vi "1.2.1-ParseYPR.vi"(9 "ASCII: VNYPR,":u8[](array[numeric])=[86, 78, 89, 80, 82, 44], 10 "Serial Byte":u8) -> (1 "Yaw":i16)   [LabVIEW 2010]
doc: "This VI parses Yaw, Pitch, and Roll (YPR) data from the VectorNav. In response to a YPR Read Request, the VectorNav will reply in the form \"$VNYPR,XX,-XXX.XX,-XXX.XX,+XXX.XX*XX\" (where X is a digit from 0-9). This string is in the form \"$<command type>,<access ID>, <yaw>,<pitch>,<roll>\".\n\nThe VI first waits for a $, then checks to make sure it has read \"VNYPR,\" correctly, then adds up each of the XX values and saves them appropriately. Since it receives these values one byte at a time , it must do some simple fixed point math to make sure the appropriate decimal value is saved."
uses:
  1.2.1-ParseYPR.ctl
panel:
  out "Heading (out)":T1 {"Yaw" format="%.19g"; "Pitch" format="%.19g"; "Roll" format="%.19g"}
  in  "Heading (in)":T1 {"Yaw" format="%.42g"; "Pitch" format="%.42g"; "Roll" format="%.42g"}
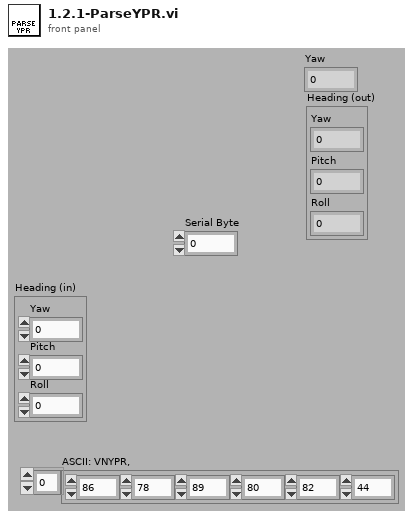
[diagram p1: front panel]
types:
  T1 = cluster{"Yaw":fxp<+/-,32,20>, "Pitch":fxp<+/-,32,20>, "Roll":fxp<+/-,32,20>}
  T2 = typedef "1.2.1-ParseYPR.ctl" = enum16{"Wait for $", "Check VNYPR", "Read numbers"}
  T3 = enum16{"Initialize", "Yaw", "Pitch", "Roll", "Done"}
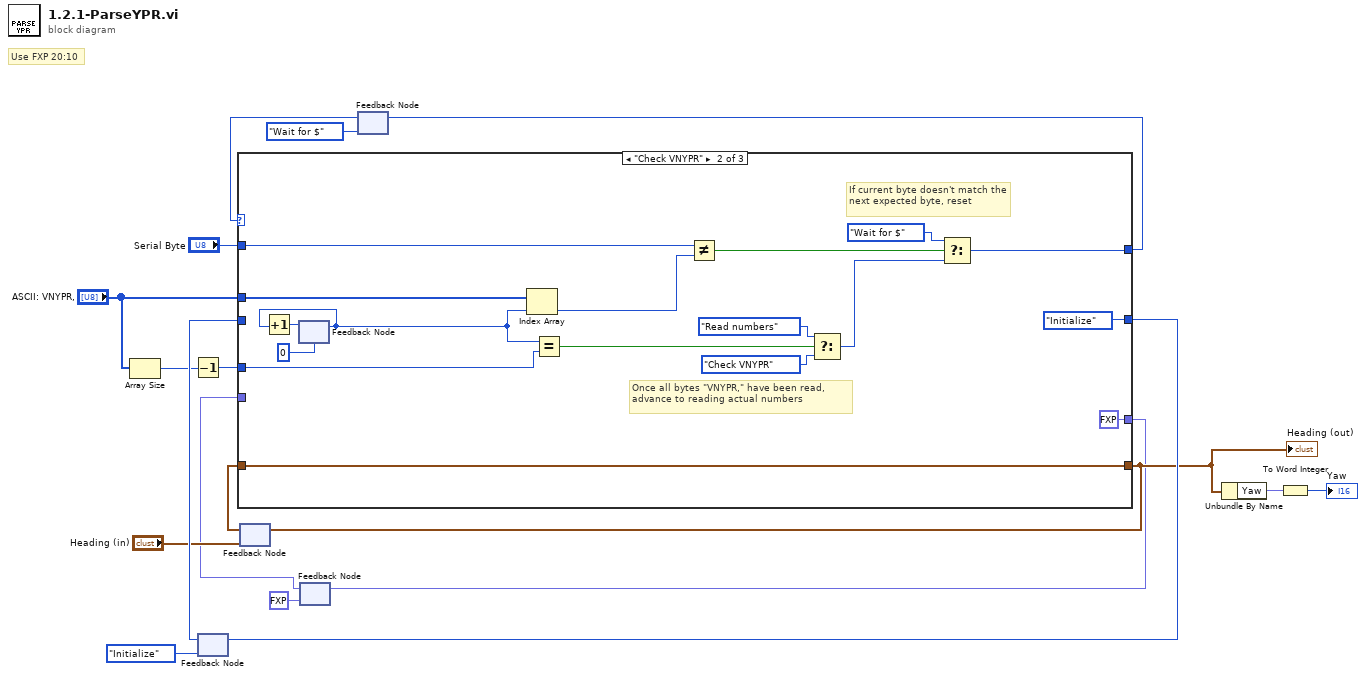
[diagram p0: block diagram]
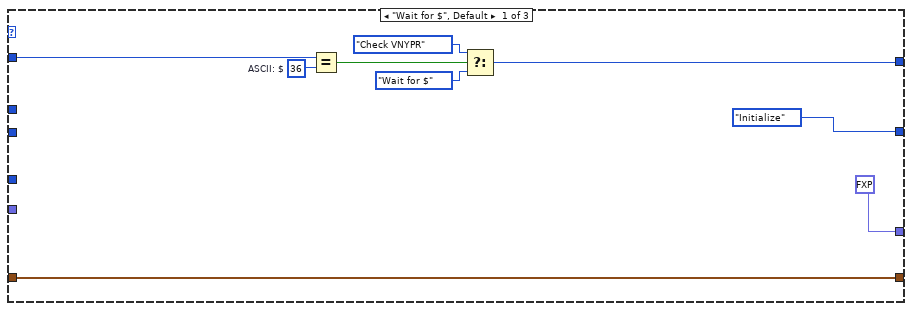
[diagram p2: hidden frame]
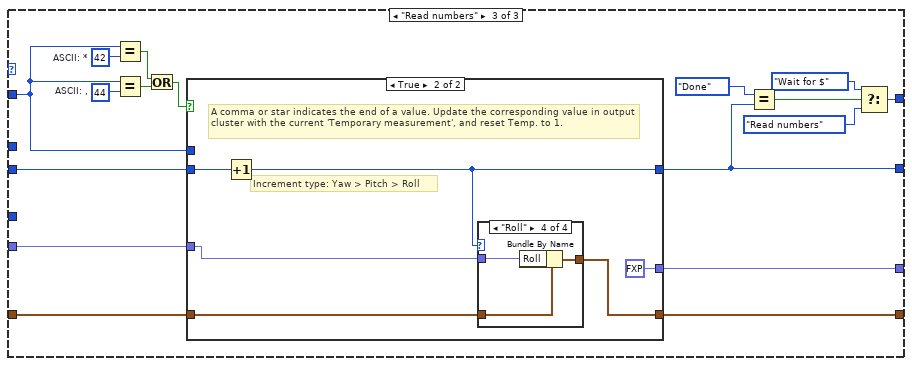
[diagram p3: hidden frame]
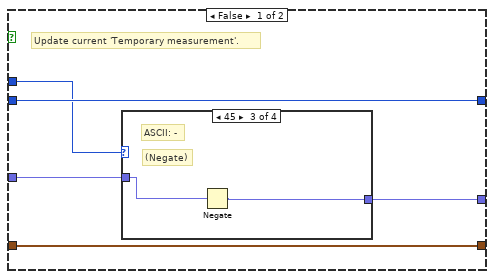
[diagram p4: hidden frame]
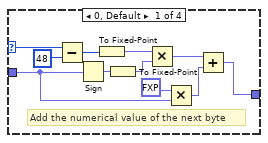
[diagram p5: hidden frame]
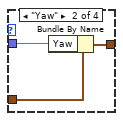
[diagram p9: hidden frame]
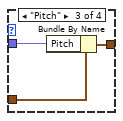
[diagram p10: hidden frame]
diagram:
  # "Use FXP 20:10"
  n1 = Array Size(array="ASCII: VNYPR,") -> (size(s)=w2:i32)
  n2 = Decrement(x=w2) -> (x-1=w1:i32)
  n3 = feedback #1(T3."Initialize" ("f")) -> (w13:T3)
  n4 = feedback #2("Heading (in)") -> (w7:T1)
  n5 = feedback #3(fxp<+/-,32,20> 1.0 ("Yaw")) -> (w5:fxp<+/-,32,20>)
  n6 = feedback #4(1.2.1-ParseYPR."Wait for $" ("1.3.1-ParseYPR")) -> (w16:T2)
  n7 = case shown="\"Check VNYPR\"" w16 {
    tunnel: [w24 w35 w49] -> w18
    tunnel: "Serial Byte" -> [w27 w41 w48]
    tunnel: [fxp<+/-,32,20> 1.0 ("Yaw") fxp<+/-,32,20> 1.0 ("Yaw") w50] -> w4
    tunnel: [w23 w42 w59] -> w6
    tunnel: w7 -> [w23 w42 w60]
    tunnel: [T3."Initialize" ("f") T3."Initialize" ("f") w57] -> w14
    tunnel: w13 -> [_ _ w58]
    tunnel: w5 -> [_ _ w45]
    tunnel: "ASCII: VNYPR," -> [_ w29 _]
    tunnel: w1 -> [_ w28 _]
    frame "Wait for $", Default {
      w26 = u8 36  # ASCII: $
      n8 = Equal?(x=w27, y=w26) -> (x = y?=w25:bool)
      n9 = Select(t=1.2.1-ParseYPR."Check VNYPR" ("1.3.1-ParseYPR"), s=w25, f=1.2.1-ParseYPR."Wait for $" ("1.3.1-ParseYPR")) -> (s? t:f=w24:T2)
    }
    frame "Check VNYPR" {
      # "If current byte doesn't match the next expected byte, reset"
      # "Once all bytes \"VNYPR,\" have been read, advance to reading actual numbers"
      n10 = feedback #5(0 ("Serial Byte")) -> (w30:i32)
      n11 = Increment(x=w30) -> (x+1=w31:i32)
      n12 = feedback-in #5(w31) -> ()
      n13 = Index Array(array=w29, index=w30) -> (element=w44:u8)
      n14 = Equal?(x=w30, y=w28) -> (x = y?=w40:bool)
      n15 = Not Equal?(x=w41, y=w44) -> (x != y?=w43:bool)
      n16 = Select(t=1.2.1-ParseYPR."Read numbers" ("1.3.1-ParseYPR"), s=w40, f=1.2.1-ParseYPR."Check VNYPR" ("1.3.1-ParseYPR")) -> (s? t:f=w33:T2)
      n17 = Select(t=1.2.1-ParseYPR."Wait for $" ("1.3.1-ParseYPR"), s=w43, f=w33) -> (s? t:f=w35:T2)
    }
    frame "Read numbers" {
      w54 = u8 42  # ASCII: *
      w61 = u8 44  # ASCII: ,
      n18 = Equal?(x=w48, y=w54) -> (x = y?=w52:bool)
      n19 = Equal?(x=w48, y=w61) -> (x = y?=w53:bool)
      n20 = Or(x=w52, y=w53) -> (x .or. y?=w51:bool)
      n21 = case shown="True" w51 {
        tunnel: w60 -> [w66 w87]
        tunnel: [w66 w86] -> w59
        tunnel: [w65 w84] -> w57
        tunnel: w58 -> [w65 w85]
        tunnel: [w63 fxp<+/-,32,20> 1.0 ("Yaw")] -> w50
        tunnel: w48 -> [w64 _]
        tunnel: w45 -> [w62 w82]
        frame False {
          # "Update current 'Temporary measurement'."
          n22 = case shown="45" w64 {
            selector: w64 -> [w76 _ _ _]
            tunnel: [w74 w78 w79 w81] -> w63
            tunnel: w62 -> [w68 w78 w80 w81]
            frame 0, Default {
              # "Add the numerical value of the next byte"
              n23 = Subtract(x=w76, y=u8 48) -> (x-y=w72:u8)
              n24 = Sign(1:w68) -> (0:w71:fxp<+/-,2,2>)
              n25 = To Fixed-Point(number=w72) -> (fixed-point=w70:fxp<+/-,32,20>)  [unwired: 1 in]
              n26 = To Fixed-Point(number=w71) -> (fixed-point=w69:fxp<+/-,32,20>)  [unwired: 1 in]
              n27 = Multiply(x=w70, y=w69) -> (x*y=w67:fxp<+/-,32,20>)
              n28 = Multiply(x=fxp<+/-,20,10> 10.0 ("Yaw"), y=w68) -> (x*y=w77:fxp<+/-,52,30>)
              n29 = Add(x=w67, y=w77) -> (x+y=w74:fxp<+/-,32,20>)
            }
            frame 43 {
              # "ASCII: +"
            }
            frame 45 {
              # "(Negate)"
              # "ASCII: -"
              n30 = Negate(x=w80) -> (-x=w79:fxp<+/-,32,20>)
            }
            frame 46 {
              # "(Ignore decimal for now)"
              # "ASCII: ."
            }
          }
        }
        frame True {
          # "Increment type: Yaw > Pitch > Roll"
          # "A comma or star indicates the end of a value. Update the corresponding value in output cluster with the current 'Temporary measurement', and reset Temp. to 1."
          n31 = Increment(x=w85) -> (x+1=w84:T3)
          n32 = case shown="\"Roll\"" w84 {
            tunnel: [w88 w91 w94 w97] -> w86
            tunnel: w87 -> [w88 w90 w93 w96]
            tunnel: w82 -> [_ w89 w92 w95]
            frame "Initialize", Default {
            }
            frame "Yaw" {
              n33 = Bundle By Name(cluster=w90, "Yaw"=w89) -> (w91:T1)
            }
            frame "Pitch" {
              n34 = Bundle By Name(cluster=w93, "Pitch"=w92) -> (w94:T1)
            }
            frame "Roll" {
              n35 = Bundle By Name(cluster=w96, "Roll"=w95) -> (w97:T1)
            }
          }
        }
      }
      n36 = Equal?(x=T3."Done", y=w57) -> (x = y?=w55:bool)
      n37 = Select(t=1.2.1-ParseYPR."Wait for $" ("1.3.1-ParseYPR"), s=w55, f=1.2.1-ParseYPR."Read numbers" ("1.3.1-ParseYPR")) -> (s? t:f=w49:T2)
    }
  }
  "Heading (out)" <- w6
  n38 = feedback-in #1(w14) -> ()
  n39 = feedback-in #2(w6) -> ()
  n40 = feedback-in #3(w4) -> ()
  n41 = feedback-in #4(w18) -> ()
  n42 = Unbundle By Name(w6) -> ("Yaw"=w10:fxp<+/-,32,20>)
  n43 = To Word Integer(number=w10) -> (16bit integer=→"Yaw":i16)
